vi "TypeDescriptor_ExtractElements.vi"(9 "Data String":string, 11 "type descriptor":i16[](array[numeric]) format="%04x") -> (0 "concatenated element descriptors":i16[](array[numeric]), 1 "Nb elements":i32, 2 "elements":T1[](array[typedef]), 3 "type descriptor dup":i16[](array[numeric]) format="%.0x")   [LabVIEW 2013, in "OpenDescriptor.lvlib"]
uses:
  OpenDescriptor.lvlib
  Descriptor Element -- cluster.ctl
  TypeDescriptor_GetPString.vi
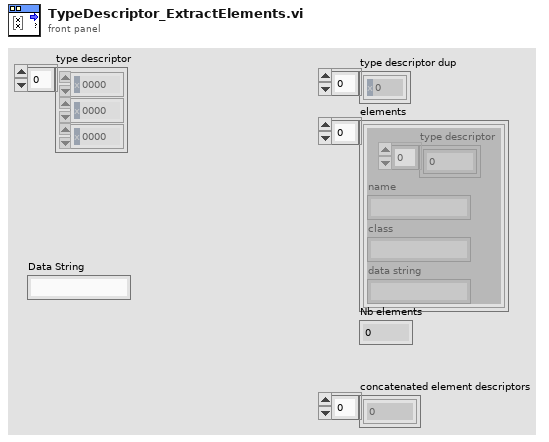
[diagram p1: front panel]
types:
  T1 = typedef "OpenDescriptor.lvlib/Descriptor Element -- cluster.ctl" = cluster{"type descriptor":i16[], "name":string, "class":string, "data string":string}
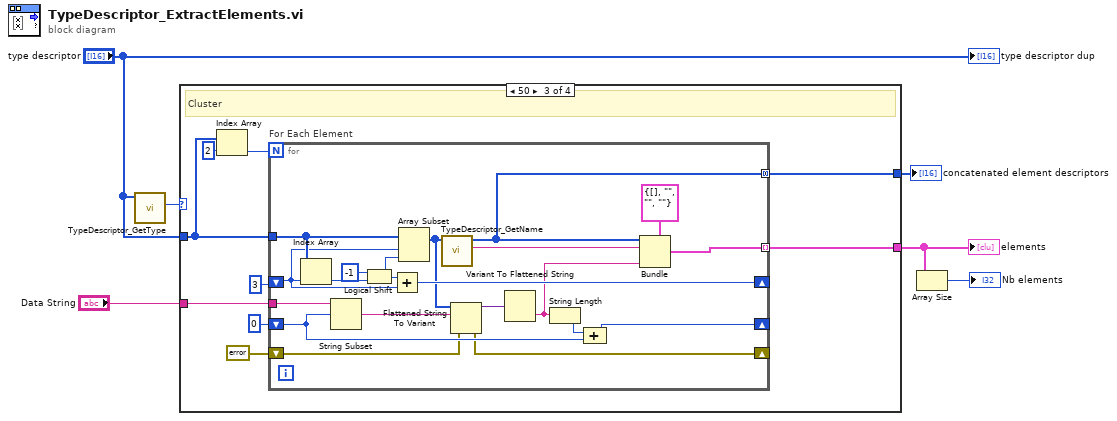
[diagram p0: block diagram]
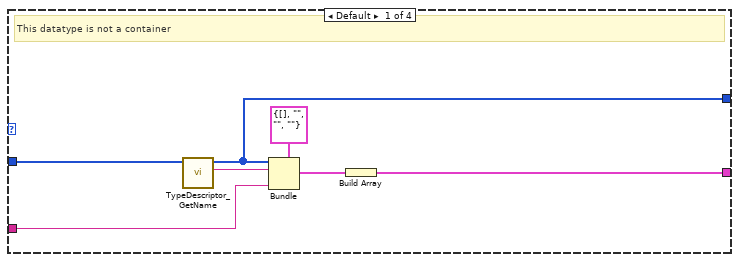
[diagram p2: hidden frame]
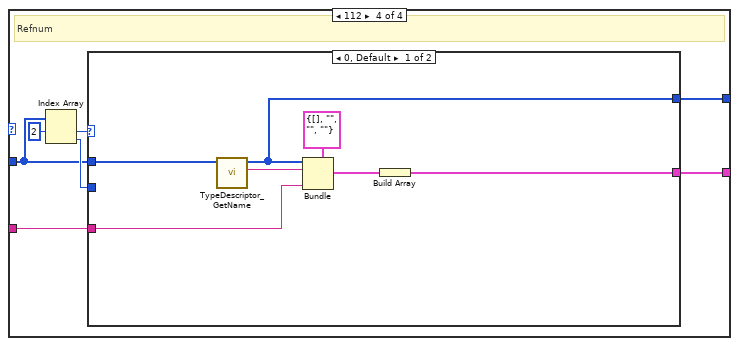
[diagram p4: hidden frame]
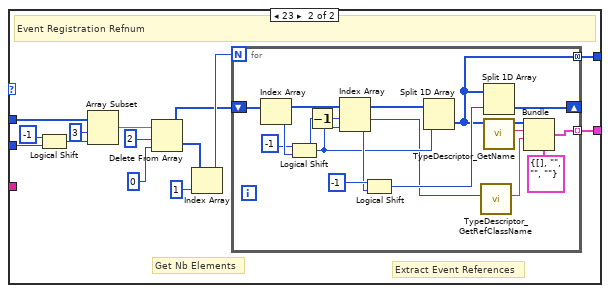
[diagram p5: hidden frame]
diagram:
  n1 = call "TypeDescriptor_GetType.vi"("type descriptor"="type descriptor") -> ("Type"=w5:u8)  [unwired: 9 in, 1 out]
  n2 = case shown="50" w5 {
    tunnel: [w9 _ w18 w45] -> w4
    tunnel: "type descriptor" -> [w11 _ w19 w46]
    tunnel: [w8 _ w17 w44] -> w2
    tunnel: "Data String" -> [w7 _ w15 w43]
    frame Default {
      # "This datatype is not a container"
      n3 = call "TypeDescriptor_GetName.vi"("type descriptor"=w11) -> ("name"=w13:string, "type descriptor dup"=w8:i16[])  [unwired: 8 in, 1 out]
      n4 = Bundle(cluster=T1 {"type descriptor"=[], "name"="", "class"="", "data string"=""} ("Descriptor Element"), "type descriptor"=w8, "name"=w13, "data string"=w7) -> (w10:T1)  [unwired: 1 in]
      n5 = Build Array(w10) -> (w9:T1[])
    }
    frame 0 {
      # "void"
    }
    frame 80 {
      # "Cluster"
      n6 = Index Array(array=w19, index=2) -> (element=w21:i16)
      n7 = for "For Each Element" {
        N: w21 -> [_]
        tunnel: w19 -> [w39]
        shift-right: [w40] -> _
        shift-left: 3 ("index") -> [w38]
        tunnel: [w35] -> w18 mode=indexing
        tunnel: [w33] -> w17 mode=concatenating
        shift-right: [w26] -> _
        shift-left: 0 -> [w27]
        tunnel: w15 -> [w32]
        shift-right: [w23] -> _
        shift-left: errorcluster {"status"=FALSE, "code"=0, "source"=""} ("error out") -> [w24]
        n8 = Index Array(array=w39, index=w38) -> (element=w41:i16)
        n9 = String Subset(string=w32, offset (0)=w27) -> (substring=w30:string)  [unwired: 1 in]
        n10 = Logical Shift(y=i16 -1, x=w41) -> (x << y=w37:i16)
        n11 = Add(x=w37, y=w38) -> (x+y=w40:i32)
        n12 = Array Subset(array=w39, index=w38, length=w37) -> (w31:i16[])
        n13 = call "TypeDescriptor_GetName.vi"("type descriptor"=w31) -> ("name"=w36:string, "type descriptor dup"=w33:i16[])  [unwired: 8 in, 1 out]
        n14 = Flattened String To Variant(4:w24, 6:w30, 7:w31) -> (0:w23:errorcluster, 3:w29:variant)
        n15 = Variant To Flattened String(Variant=w29) -> (data string=w25:string)  [unwired: 1 out]
        n16 = String Length(string=w25) -> (length=w28:i32)
        n17 = Compound Arithmetic op=ADD(w28, w27) -> (w26:i32)
        n18 = Bundle(cluster=T1 {"type descriptor"=[], "name"="", "class"="", "data string"=""} ("Descriptor Element"), "type descriptor"=w33, "name"=w36, "data string"=w25) -> (w35:T1)  [unwired: 1 in]
      }
    }
    frame 112 {
      # "Refnum"
      n19 = Index Array(array=w46, index #1=2 ("index")) -> (element #1=w48:i16, element #2=w47:i16)  [unwired: 1 in]
      n20 = case shown="0, Default" w48 {
        tunnel: w47 -> [_ w67]
        tunnel: w46 -> [w53 w70]
        tunnel: [w51 w58] -> w45
        tunnel: [w52 w57] -> w44
        tunnel: w43 -> [w50 _]
        frame 0, Default {
          n21 = call "TypeDescriptor_GetName.vi"("type descriptor"=w53) -> ("name"=w54:string, "type descriptor dup"=w52:i16[])  [unwired: 8 in, 1 out]
          n22 = Bundle(cluster=T1 {"type descriptor"=[], "name"="", "class"="", "data string"=""} ("Descriptor Element"), "type descriptor"=w52, "name"=w54, "data string"=w50) -> (w56:T1)  [unwired: 1 in]
          n23 = Build Array(w56) -> (w51:T1[])
        }
        frame 23 {
          # "Extract Event References"
          # "Get Nb Elements"
          # "Event Registration Refnum"
          n24 = Logical Shift(y=i16 -1, x=w67) -> (x << y=w66:i16)
          n25 = Array Subset(array=w70, index=3, length=w66) -> (w65:i16[])
          n26 = Delete From Array(array=w65, length=2 ("index"), index=0) -> (deleted portion=w63:i16[], array with subset deleted=w59:i16[])
          n27 = Index Array(array=w63, index=1) -> (element=w60:i16)
          n28 = for {
            N: w60 -> [_]
            shift-right: [w78] -> _
            shift-left: w59 -> [w81]
            tunnel: [w73] -> w58 mode=indexing
            tunnel: [w71] -> w57 mode=concatenating
            n29 = Index Array(array=w81) -> (element=w86:i16)  [unwired: 1 in]
            n30 = Logical Shift(y=i16 -1, x=w86) -> (x << y=w80:i16)
            n31 = Decrement(x=w80) -> (x-1=w82:i16)
            n32 = Index Array(array=w81, index #1=w82, index #2=w80) -> (element #1=w77:i16, element #2=w83:i16)
            n33 = Logical Shift(y=i16 -1, x=w83) -> (x << y=w79:i16)
            n34 = Split 1D Array(array=w81, index=w80) -> (second subarray=w71:i16[])  [unwired: 1 out]
            n35 = call "TypeDescriptor_GetRefClassName.vi"("Ref Class"=w77) -> ("Reference Class"=w75:string)  [unwired: 10 in]
            n36 = Split 1D Array(array=w71, index=w79) -> (second subarray=w78:i16[])  [unwired: 1 out]
            n37 = call "TypeDescriptor_GetName.vi"("type descriptor"=w71) -> ("name"=w74:string, "type descriptor dup"=w76:i16[])  [unwired: 8 in, 1 out]
            n38 = Bundle(cluster=T1 {"type descriptor"=[], "name"="", "class"="", "data string"=""} ("Descriptor Element"), "type descriptor"=w76, "name"=w74, "class"=w75) -> (w73:T1)  [unwired: 1 in]
          }
        }
      }
    }
  }
  "elements" <- w4
  "concatenated element descriptors" <- w2
  n39 = Array Size(array=w4) -> (size(s)=→"Nb elements":i32)
  "type descriptor dup" <- "type descriptor"
